vi "SEM shutter.vi"(4 "Specimen I spike threshold (nA)":sgl=0.005, 5 "Retry #":i32=3, 6 "Shutter close":bool, 7 "delay (ms)":u32=1000, 8 "Shutter AO4":tag="Log/ao3", 9 "Shutter AO3":tag="Log/ao2", 10 "Shutter AO2":tag="Log/ao1", 11 "Shutter AO1":tag="Log/ao0") -> (0 "error out":errorcluster, 1 "Shutter close feedback":bool, 2 "Fail #":u8, 3 "SEM shutter status":string)   [LabVIEW 2012]
uses:
  <vilib>/DAQmx/write.llb/DAQmx Write (Analog 1D DBL NChan 1Samp).vi
  <vilib>/DAQmx/create/channels.llb/DAQmx Create Channel (AO-Voltage-Basic).vi
  <vilib>/DAQmx/miscellaneous.llb/DAQmx Fill In Error Info.vi
  <vilib>/gmath/NI_Gmath.lvlib
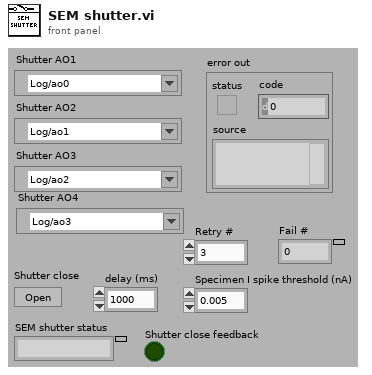
[diagram p1: front panel]
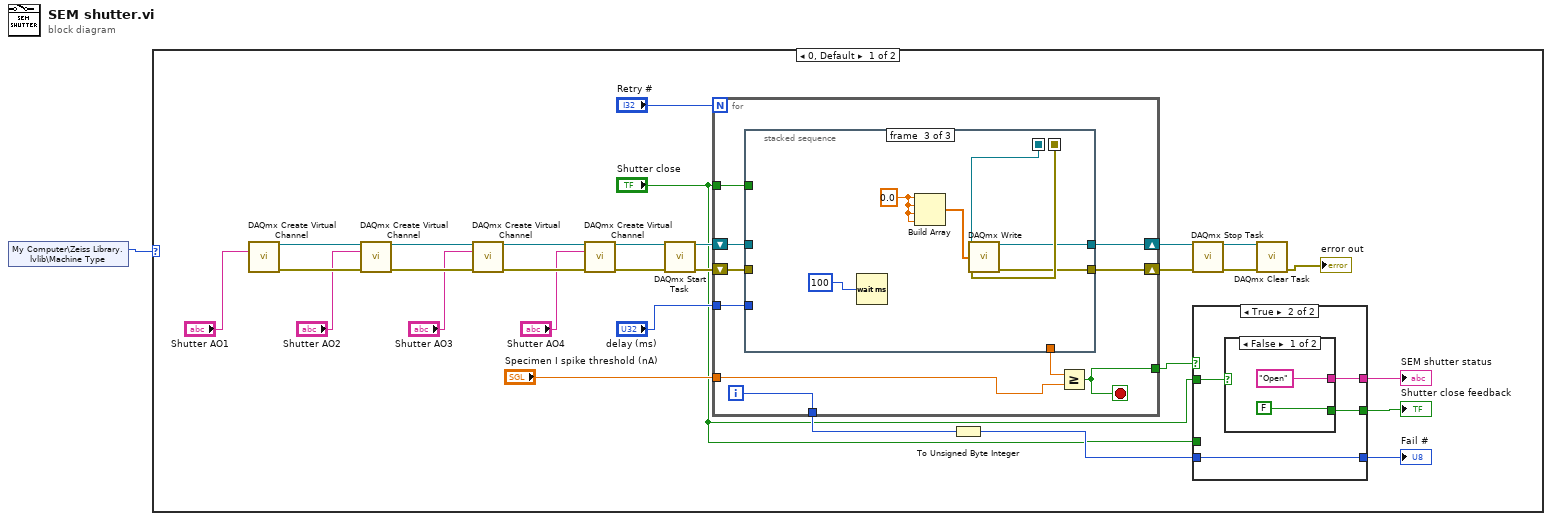
[diagram p0: block diagram]
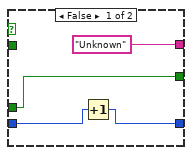
[diagram p2: hidden frame]
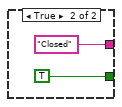
[diagram p3: hidden frame]
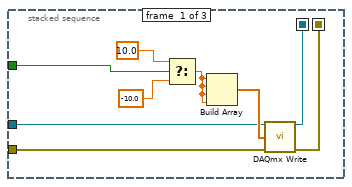
[diagram p4: hidden frame]
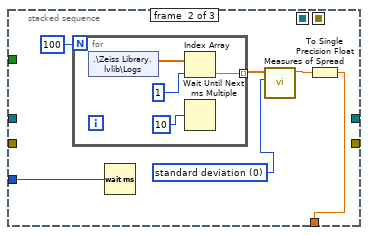
[diagram p5: hidden frame]
diagram:
  n1 = shared-variable "My Computer\\Zeiss Library.lvlib\\Machine Type"() -> (w1:u8)  [unwired: 1 in, 1 out]
  n2 = case shown="0, Default" w1 {
    frame 0, Default {
      n3 = call-poly <vilib>:"DAQmx Create Virtual Channel.vi"("physical channels"="Shutter AO1") -> ("task out"=w19:refnum<k21>, "error out"=w20:errorcluster)  [unwired: 13 in]
      n4 = call-poly <vilib>:"DAQmx Create Virtual Channel.vi"("task in"=w19, "physical channels"="Shutter AO2", "error in"=w20) -> ("task out"=w25:refnum<k21>, "error out"=w26:errorcluster)  [unwired: 11 in]
      n5 = call-poly <vilib>:"DAQmx Create Virtual Channel.vi"("task in"=w25, "physical channels"="Shutter AO3", "error in"=w26) -> ("task out"=w23:refnum<k21>, "error out"=w24:errorcluster)  [unwired: 11 in]
      n6 = call-poly <vilib>:"DAQmx Create Virtual Channel.vi"("task in"=w23, "physical channels"="Shutter AO4", "error in"=w24) -> ("task out"=w14:refnum<k21>, "error out"=w13:errorcluster)  [unwired: 11 in]
      n7 = call <vilib>:"DAQmx Start Task.vi"("task/channels in"=w14, "error in"=w13) -> ("task out"=w12:refnum<k21>, "error out"=w11:errorcluster)  [unwired: 12 in]
      n8 = for {
        N: "Retry #" -> [_]
        shift-right: [w52] -> w16
        shift-left: w12 -> [w51]
        shift-right: [w50] -> w15
        shift-left: w11 -> [w49]
        tunnel: "Shutter close" -> [w47]
        tunnel: [w46] -> w8
        tunnel: [w45] -> w6
        tunnel: "Specimen I spike threshold (nA)" -> [w44]
        tunnel: "delay (ms)" -> [w43]
        i -> [w45]
        stop <- w46 stop-if-true
        n9 = stacked-sequence {
          seq-local: [w61 _ _] -> [_ _ w76]
          seq-local: [w60 _ _] -> [_ _ w75]
          tunnel: [_ _ w74] -> w52
          tunnel: [_ _ w73] -> w50
          tunnel: w51 -> [w55 _ _]
          tunnel: w49 -> [w54 _ _]
          tunnel: [_ w65 _] -> w48
          tunnel: w47 -> [w53 _ _]
          tunnel: w43 -> [_ w62 _]
          frame #0 {
            n10 = Select(t=10.0, s=w53, f=-10.0) -> (s? t:f=w56:dbl)
            n11 = Build Array(w56, w56, w56, w56) -> (w57:dbl[])
            n12 = call-poly <vilib>:"DAQmx Write.vi"("task/channels in"=w55, "data"=w57, "error in"=w54) -> ("task out"=w61:refnum<k21>, "error out"=w60:errorcluster)  [unwired: 10 in, 1 out]
          }
          frame #1 {
            w63 = 0 items=["standard deviation", "range", "mean absolute deviation", "interquartile range"] ("type")
            n13 = for {
              N: 100 -> [_]
              tunnel: [w69] -> w67 mode=indexing
              n14 = shared-variable ".\\Zeiss Library.lvlib\\Logs"() -> (w71:sgl[])  [unwired: 1 in, 1 out]
              n15 = Index Array(array=w71, index=1) -> (element=w69:sgl)
              n16 = Wait Until Next ms Multiple(millisecond multiple=u32 10) -> ()  [unwired: 1 out]
            }
            n17 = Wait (ms)(milliseconds to wait=w62) -> ()  [unwired: 1 out]
            n18 = call <vilib>:"Measures of Spread.vi"("type"=w63, "x array"=w67) -> ("spread value"=w64:dbl)  [unwired: 8 in, 1 out]
            n19 = To Single Precision Float(number=w64) -> (single precision float=w65:sgl)
          }
          frame #2 {
            w77 = 0.0 ("element")
            n20 = Wait (ms)(milliseconds to wait=u32 100) -> ()  [unwired: 1 out]
            n21 = Build Array(w77, w77, w77, w77) -> (w78:dbl[])
            n22 = call-poly <vilib>:"DAQmx Write.vi"("task/channels in"=w76, "data"=w78, "error in"=w75) -> ("task out"=w74:refnum<k21>, "error out"=w73:errorcluster)  [unwired: 10 in, 1 out]
          }
        }
        n23 = Greater Or Equal?(x=w48, y=w44) -> (x >= y?=w46:bool)
      }
      n24 = To Unsigned Byte Integer(number=w6) -> (unsigned 8bit integer=w4:u8)
      n25 = call <vilib>:"DAQmx Stop Task.vi"("task/channels in"=w16, "error in"=w15) -> ("task out"=w29:refnum<k21>, "error out"=w30:errorcluster)  [unwired: 12 in]
      n26 = case shown="True" w8 {
        tunnel: "Shutter close" -> [_ w38]
        tunnel: ["Unknown" w37] -> w7
        tunnel: [w33 w36] -> w5
        tunnel: w4 -> [w32 w36]
        tunnel: [w31 w35] -> w2
        tunnel: "Shutter close" -> [w31 _]
        frame False {
          n27 = Increment(x=w32) -> (x+1=w33:u8)
        }
        frame True {
          n28 = case shown="False" w38 {
            tunnel: ["Open" "Closed"] -> w37
            tunnel: [FALSE ("Shutter close") TRUE ("Shutter close")] -> w35
            frame False {
            }
            frame True {
            }
          }
        }
      }
      "Fail #" <- w5
      "SEM shutter status" <- w7
      "Shutter close feedback" <- w2
      n29 = call <vilib>:"DAQmx Clear Task.vi"("task in"=w29, "error in"=w30) -> ("error out"=→"error out":errorcluster)  [unwired: 13 in]
    }
    frame 1 {
    }
  }
